vi "Regulation_Combined.vi"(4 "k_d":dbl, 5 "Coerce?":bool, 6 "k_i":dbl, 7 "DATA":dbl, 9 "k_p":dbl, 10 "SP":dbl, 11 "Regulation type":T1(ring)) -> (0 "D":dbl, 1 "I":dbl, 2 "P":dbl, 3 "u":dbl)   [LabVIEW 2022 SP3]
uses:
  ID_Regulering.vi
  P_regulering.vi
  PI_Regulering.vi
  PD_Regulering.vi
  PID_Regulering.vi
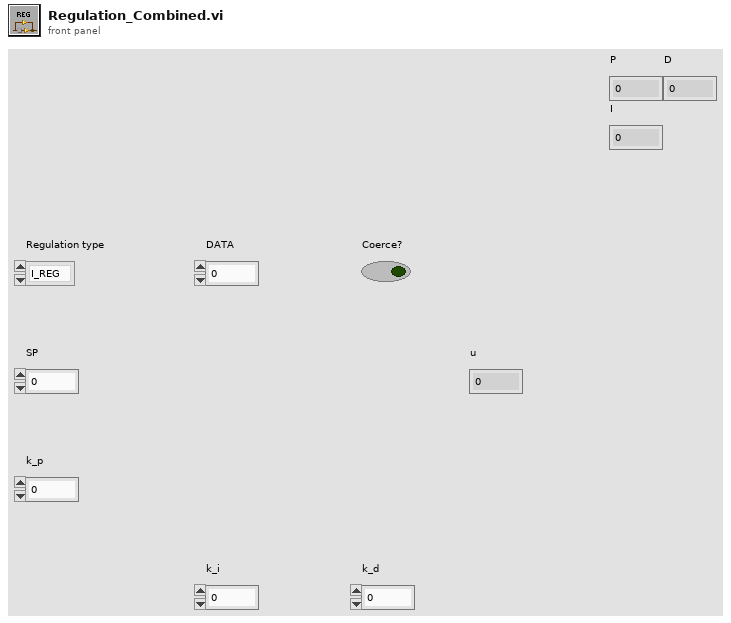
[diagram p1: front panel]
types:
  T1 = enum16{"I_REG", "ID_REG", "P_REG", "PI_REG", "PD_REG", "PID_REG"}
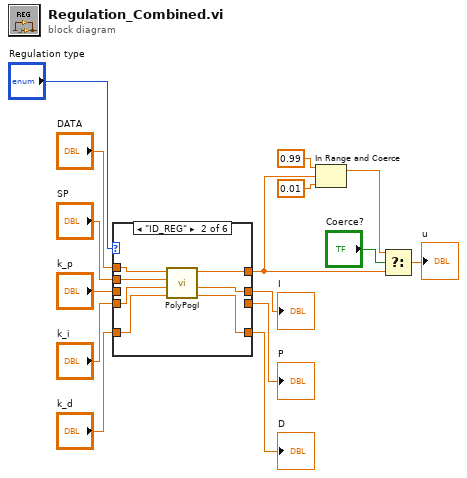
[diagram p0: block diagram]
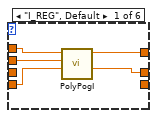
[diagram p2: hidden frame]
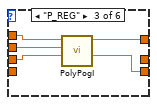
[diagram p3: hidden frame]
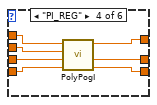
[diagram p4: hidden frame]
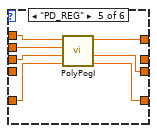
[diagram p5: hidden frame]
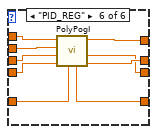
[diagram p6: hidden frame]
diagram:
  n1 = case shown="\"ID_REG\"" "Regulation type" {
    tunnel: "DATA" -> [w18 w27 w32 w39 w46 w55]
    tunnel: [w20 w23 w29 w35 w42 w50] -> w12
    tunnel: "SP" -> [w19 w26 w31 w38 w45 w54]
    tunnel: "k_i" -> [w17 w25 _ w36 _ w52]
    tunnel: "k_p" -> [_ _ w30 w37 w44 w53]
    tunnel: "k_d" -> [_ w24 _ _ w43 w51]
    tunnel: [w16 w22 _ w34 _ w48] -> w3
    tunnel: [_ w21 _ _ w40 w49] -> w2
    tunnel: [_ _ w28 w33 w41 w47] -> w1
    frame "I_REG", Default {
      n2 = call-poly "PolyPogI.vi"("k_i"=w17, "SP"=w19, "DATA"=w18) -> ("i_id"=w16:dbl, "u_id"=w20:dbl)  [unwired: 5 in, 2 out]
    }
    frame "ID_REG" {
      n3 = call-poly "PolyPogI.vi"("k_d"=w24, "k_i"=w25, "SP"=w26, "DATA"=w27) -> ("d_id"=w21:dbl, "i_id"=w22:dbl, "u_id"=w23:dbl)  [unwired: 4 in, 1 out]
    }
    frame "P_REG" {
      n4 = call-poly "PolyPogI.vi"("k_p"=w30, "SP"=w31, "DATA"=w32) -> ("p_p"=w28:dbl, "u_p"=w29:dbl)  [unwired: 6 in, 1 out]
    }
    frame "PI_REG" {
      n5 = call-poly "PolyPogI.vi"("k_i"=w36, "k_p"=w37, "SP"=w38, "DATA"=w39) -> ("p_pi"=w33:dbl, "i_pi"=w34:dbl, "u_pi"=w35:dbl)  [unwired: 4 in, 1 out]
    }
    frame "PD_REG" {
      n6 = call-poly "PolyPogI.vi"("k_d"=w43, "k_p"=w44, "SP"=w45, "DATA"=w46) -> ("d_pd"=w40:dbl, "p_pd"=w41:dbl, "u_pd"=w42:dbl)  [unwired: 4 in, 1 out]
    }
    frame "PID_REG" {
      n7 = call-poly "PolyPogI.vi"("k_d"=w51, "k_i"=w52, "k_p"=w53, "SP"=w54, "DATA"=w55) -> ("i_pid"=w48:dbl, "p_pid"=w47:dbl, "u_pid"=w50:dbl, "d_pid"=w49:dbl)  [unwired: 2 in, 1 out]
    }
  }
  "P" <- w1
  "I" <- w3
  "D" <- w2
  n8 = In Range and Coerce(upper limit=0.99, x=w12, lower limit=0.01) -> (coerced(x)=w13:dbl)  [unwired: 1 out]
  n9 = Select(t=w13, s="Coerce?", f=w12) -> (s? t:f=→"u":dbl)
